vi "real time imaging v1.vi"() -> ()   [LabVIEW 2016]
uses:
  C:/Laser generated ultrasound/Labview/Kinesis Control/Thorlabs.MotionControl.Controls.dll
  Thorlabs.MotionControl.Controls.dll
  C:/Laser generated ultrasound/Labview/Kinesis Control/Thorlabs.MotionControl.KCube.BrushlessMotorCLI.dll
  Thorlabs.MotionControl.KCube.BrushlessMotorCLI.dll
  <vilib>/Analysis/3filter.llb/Filter Passband Type.ctl
  <vilib>/Analysis/baseanly.llb/Mean (DBL).vi
  <vilib>/Analysis/baseanly.llb/Real A x B.vi
  <vilib>/Utility/file.llb/Write To Spreadsheet File (DBL).vi
  <instrlib>/niScope/Acquire/Fetch/niScope Fetch.vi
  <vilib>/Analysis/Matrix/Numeric/Conversions/Array To Matrix - RA2.vi
  <vilib>/Analysis/Matrix/Numeric/Conversions/Matrix To Array - RM.vi
  <vilib>/Analysis/3filter.llb/Butterworth Filter (DBL).vi
  <instrlib>/niScope/Acquire/Fetch/niScope Multi Fetch.vi
  <vilib>/Analysis/NI_AALBase.lvlib
  <vilib>/Analysis/Matrix/NI_Matrix.lvlib
  <vilib>/Analysis/NI_AALPro.lvlib
panel:
  in  "stop":bool
  in  "Tab Control":T1(tab)
  in  "File Location":string="C:\\Laser generated ultrasound\\Labview\\Kinesis Control\\test data"
  in  "File name":string="scan_1"
  in  "SerialNumber":string="28251512"
  in  "Scan Length (mm)":dbl=20.0
  in  "Pullback speed (mm/s)":dbl=40.0
  in  "Repetition rate (Hz)":dbl=100.0
  in  "vertical range (V)":dbl=0.5 min=0.0 max=10.0 step=0.5
  in  "Depth (mm)":i32=15
  in  "Start acquisition":bool
  out "Number of samples":dbl
  out "number of a-lines":dbl
  in  "Apply frequency filter":bool
  in  "High Cutoff (MHz)":dbl=45.0
  in  "Low Cutoff (MHz)":dbl=1.0
  in  "Number of points":i32=150
  in  "Exponent":dbl=2.5
  out "?":cluster{dbl[], dbl[]}(graph)
  in  "Preview A-line?":bool
  in  "Start save":bool
  out "Intensity Graph":dbl[][](graph)
  in  "Stop save":bool
  out "Acquiring Data":bool
  in  "KCubeBrushlessControl":refnum<k24>(container)
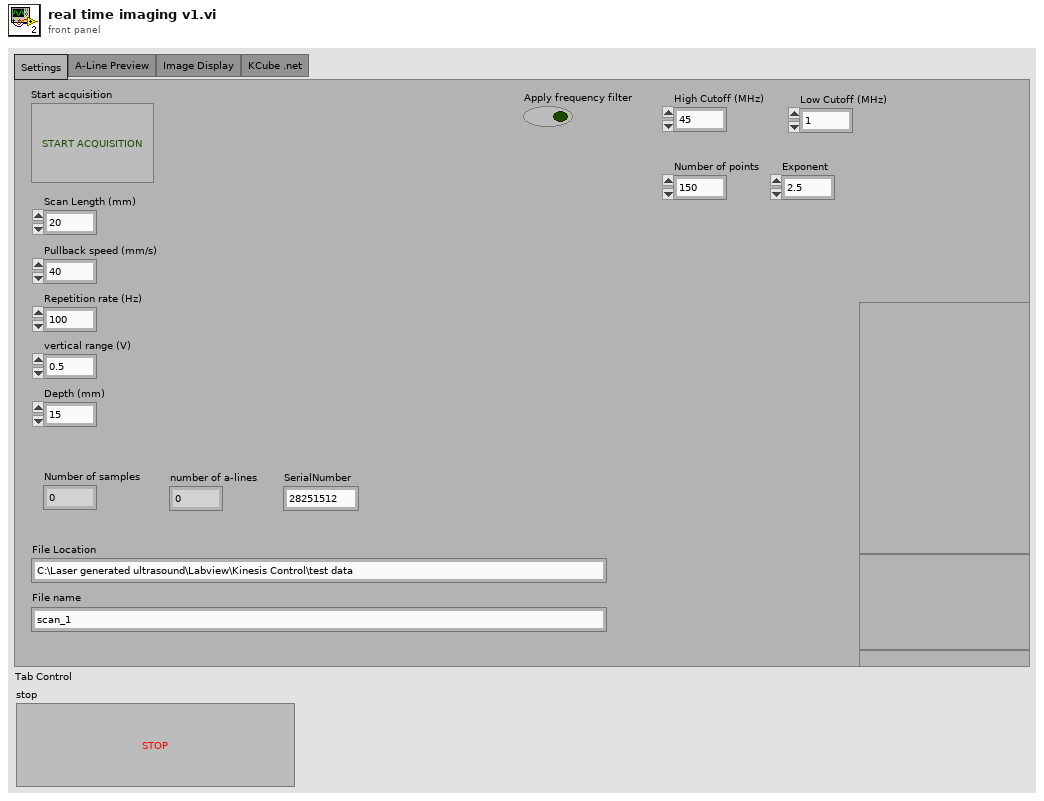
[diagram p1: front panel]
types:
  T1 = enum32{"Settings", "A-Line Preview", "Image Display", "KCube .net"}
  T2 = typedef "NI_AALBase.lvlib/Filter Passband Type.ctl" = enum32{"Lowpass", "Highpass", "Bandpass", "Bandstop"}
  T3 = typedef "NI_Matrix.lvlib/RealMatrix.ctl" = dbl[][]
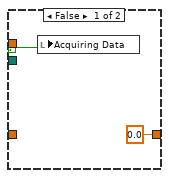
[diagram p8: hidden frame]
diagram:
  n1 = flat-sequence {
    tunnel: [w112] -> w71
    tunnel: [w111] -> w69
    tunnel: [w110] -> w67
    tunnel: [w108] -> w65
    tunnel: [w107] -> w63
    tunnel: [w95] -> w61
    tunnel: [w96] -> w59
    tunnel: ["Scan Length (mm)"] -> w57
    tunnel: ["Pullback speed (mm/s)"] -> w55
    tunnel: [w79] -> w53
    tunnel: ["File Location"] -> w52
    tunnel: ["File name"] -> w51
    tunnel: [w88] -> w43
    tunnel: [w88] -> w40
    tunnel: [w81] -> w10
    tunnel: ["Depth (mm)"] -> w5
    tunnel: [w79] -> w4
    tunnel: [w74] -> w3
    tunnel: [w73] -> w2
    tunnel: [w72] -> w1
    tunnel: w71 -> [w175]
    tunnel: [w175] -> w70
    tunnel: w69 -> [w174]
    tunnel: [w174] -> w68
    tunnel: w67 -> [w173]
    tunnel: [w173] -> w66
    tunnel: w65 -> [w172]
    tunnel: [w172] -> w64
    tunnel: w63 -> [w171]
    tunnel: [w171] -> w62
    tunnel: w61 -> [w170]
    tunnel: [w170] -> w60
    tunnel: w59 -> [w169]
    tunnel: [w169] -> w58
    tunnel: w57 -> [w168]
    tunnel: [w168] -> w56
    tunnel: w55 -> [w167]
    tunnel: [w167] -> w54
    tunnel: w53 -> [w165]
    tunnel: w52 -> [w135]
    tunnel: w51 -> [w134]
    tunnel: w43 -> [w142]
    tunnel: [w142] -> w42
    tunnel: w40 -> [w140]
    tunnel: w10 -> [_]
    tunnel: [w128] -> w9
    tunnel: w5 -> [w132]
    tunnel: w4 -> [w131]
    tunnel: w3 -> [w127]
    tunnel: w2 -> [w126]
    tunnel: w1 -> [w125]
    tunnel: w70 -> [w188]
    tunnel: w68 -> [w183]
    tunnel: w66 -> [w184]
    tunnel: [w188] -> w50
    tunnel: [w183] -> w49
    tunnel: [w184] -> w48
    tunnel: w64 -> [w182]
    tunnel: w62 -> [w181]
    tunnel: [w182] -> w47
    tunnel: [w181] -> w46
    tunnel: [w180] -> w45
    tunnel: w60 -> [w179]
    tunnel: [w179] -> w44
    tunnel: w58 -> [w180]
    tunnel: w56 -> [_]
    tunnel: w54 -> [w178]
    tunnel: w42 -> [w177]
    tunnel: [w177] -> w41
    tunnel: w9 -> [w176]
    tunnel: [w176] -> w8
    tunnel: w50 -> [w201]
    tunnel: [w201] -> w39
    tunnel: w49 -> [w200]
    tunnel: [w200] -> w37
    tunnel: w48 -> [w199]
    tunnel: [w199] -> w35
    tunnel: w47 -> [w198]
    tunnel: [w197] -> w33
    tunnel: w46 -> [w196]
    tunnel: [w195] -> w31
    tunnel: w45 -> [w194]
    tunnel: [w191] -> w29
    tunnel: w44 -> [w193]
    tunnel: [w190] -> w27
    tunnel: w41 -> [w192]
    tunnel: w8 -> [w189]
    tunnel: [w189] -> w7
    tunnel: w39 -> [w231]
    tunnel: [w231] -> w38
    tunnel: w37 -> [w230]
    tunnel: [w230] -> w36
    tunnel: w35 -> [w229]
    tunnel: [w229] -> w34
    tunnel: w33 -> [w228]
    tunnel: [w228] -> w32
    tunnel: w31 -> [w227]
    tunnel: [w227] -> w30
    tunnel: w29 -> [w226]
    tunnel: [w224] -> w28
    tunnel: w27 -> [w225]
    tunnel: [w223] -> w26
    tunnel: [w219] -> w25
    tunnel: w7 -> [w218]
    tunnel: [w218] -> w6
    tunnel: w38 -> [w243]
    tunnel: w36 -> [w241]
    tunnel: w34 -> [w242]
    tunnel: [w243] -> w24
    tunnel: [w241] -> w22
    tunnel: [w242] -> w20
    tunnel: w32 -> [w240]
    tunnel: w30 -> [w239]
    tunnel: [w240] -> w18
    tunnel: [w239] -> w16
    tunnel: [w235] -> w14
    tunnel: [w234] -> w12
    tunnel: w28 -> [w238]
    tunnel: w26 -> [w237]
    tunnel: w25 -> [w236]
    tunnel: w6 -> [w233]
    tunnel: w24 -> [w526]
    tunnel: [w526] -> w23
    tunnel: w22 -> [w525]
    tunnel: [w525] -> w21
    tunnel: w20 -> [w524]
    tunnel: [w524] -> w19
    tunnel: w18 -> [w523]
    tunnel: [w523] -> w17
    tunnel: w16 -> [w522]
    tunnel: [w522] -> w15
    tunnel: w14 -> [w521]
    tunnel: [w521] -> w13
    tunnel: w12 -> [w520]
    tunnel: [w520] -> w11
    tunnel: w23 -> [w528]
    tunnel: w21 -> [w527]
    tunnel: w19 -> [_]
    tunnel: w17 -> [w532]
    tunnel: w15 -> [w531]
    tunnel: w13 -> [w530]
    tunnel: w11 -> [w529]
    frame #0 {
      # "add extra a-lines as a buffer"
      # "calculate number of a-lines"
      # "Initiialise data array"
      # "round trip"
      # "speed of sound"
      # "convert depth to samples"
      # "convert to metre"
      # "Intialise all the equipment\n1. Motor\n2. Trigger\n3. Acquisition"
      n2 = Multiply(x=1500 ("y"), y=1e-08) -> (x*y=w100:dbl)
      n3 = local read "Pullback speed (mm/s)"() -> (w85:dbl)
      n4 = local read "Scan Length (mm)"() -> (w86:dbl)
      n5 = call "pulse_init.vi"("Repetition rate"="Repetition rate (Hz)") -> ("error out"=w107:errorcluster, "Refnum out"=w108:refnum<k21>)  [unwired: 9 in]
      n6 = local read "Repetition rate (Hz)"() -> (w84:dbl)
      n7 = Divide(x="Depth (mm)", y=1000) -> (x/y=w99:dbl)
      n8 = Multiply(x=w99, y=2.0) -> (x*y=w97:dbl)
      n9 = property class="KCubeBrushlessControl"(reference="KCubeBrushlessControl", "SerialNumber"="SerialNumber") -> (reference out=w116:refnum<k24>, error out=w115:errorcluster)  [unwired: 1 in]
      n10 = Divide(x=w97, y=w100) -> (x/y=w102:dbl)
      n11 = local read "Scan Length (mm)"() -> (w75:dbl)
      n12 = local read "Pullback speed (mm/s)"() -> (w73:dbl)
      n13 = Round Toward +Infinity(x=w102) -> (ceil(x): smallest int >= x=w79:dbl)
      "Number of samples" <- w79
      n14 = Initialize Array(0.0 ("element"), w79) -> (w89:dbl[])
      n15 = for {
        N: w79 -> [_]
        shift-right: [w124] -> w88
        shift-left: w89 -> [w123]
        i -> [w122]
        # "Create time axis"
        n16 = To Double Precision Float(number=w122) -> (double precision float=w121:dbl)
        n17 = Multiply(x=w121, y=1e-08) -> (x*y=w119:dbl)
        n18 = Replace Array Subset(array=w123, new element=w119, index=w122) -> (w124:dbl[])
      }
      n19 = Divide(x=w86, y=w85) -> (x/y=w83:dbl)
      n20 = local read "Repetition rate (Hz)"() -> (w72:dbl)
      n21 = Multiply(x=w83, y=w84) -> (x*y=w82:dbl)
      n22 = call "scope_init.vi"("Num Samples"=w79, "vertical range"="vertical range (V)", "Averages"=1) -> ("error out"=w95:errorcluster, "IVI Refnum out"=w96:refnum<k15>)  [unwired: 7 in]
      n23 = Initialize Array(0.0 ("element"), w79, w82) -> (w81:dbl[][])
      n24 = invoke class="KCubeBrushlessControl" method="CreateDevice"(reference=w116, error in=w115) -> (reference out=w114:refnum<k24>, error out=w113:errorcluster)  [unwired: 1 in, 1 out]
      n25 = Divide(x=w73, y=w72) -> (x/y=w76:dbl)
      n26 = Divide(x=w75, y=w76) -> (x/y=w77:dbl)
      n27 = Add(x=w77, y=0.0) -> (x+y=w74:dbl)
      "number of a-lines" <- w74
      n28 = property class="KCubeBrushlessControl"(reference=w114, error in=w113) -> (reference out=w112:refnum<k24>, error out=w111:errorcluster, "Device"=w110:refnum<k24>)
    }
    frame #1 {
      w143 = "\r"
      w146 = "\t"
      # "Save the header file"
      # "Initialise the data matrix"
      # "Initialise the data matrix\nSave the Header file"
      n29 = local read "Repetition rate (Hz)"() -> (w152:dbl)
      n30 = local read "Number of samples"() -> (w158:dbl)
      n31 = local read "number of a-lines"() -> (w155:dbl)
      n32 = local read "Scan Length (mm)"() -> (w149:dbl)
      n33 = local read "Pullback speed (mm/s)"() -> (w145:dbl)
      n34 = Number To Decimal String(number=w158) -> (decimal integer string=w157:string)  [unwired: 1 in]
      n35 = Number To Decimal String(number=w152) -> (decimal integer string=w151:string)  [unwired: 1 in]
      n36 = Number To Decimal String(number=w155) -> (decimal integer string=w154:string)  [unwired: 1 in]
      n37 = Number To Decimal String(number=w149) -> (decimal integer string=w148:string)  [unwired: 1 in]
      n38 = Concatenate Strings(w135, "\\" ("string"), w134, "_hdr.txt" ("string")) -> (w163:string)
      n39 = Divide(x=w132, y=w131) -> (x/y=w130:dbl)
      n40 = Number To Decimal String(number=w145) -> (decimal integer string=w144:string)  [unwired: 1 in]
      n41 = Concatenate Strings(w135, "\\" ("string"), w134, "_taxis.txt" ("string")) -> (w139:string)
      n42 = Divide(x=w126, y=w125) -> (x/y=w133:dbl)
      n43 = String To Path(string=w139) -> (path=w136:path)
      n44 = property on="Intensity Graph" class="IntGraph (strict)"("XScale.Multiplier"=w133, "YScale.Multiplier"=w130) -> ()  [unwired: 2 in, 2 out]
      n45 = property on="Intensity Graph" class="IntGraph (strict)"("ZScale.MarkerVals[]"=cluster{dbl, u32}[] [{0.0, 0}, {25.0, 16711680}, {50.0, 16744192}, {75.0, 16777087}, {100.0, 16777215}] ("Z Scale.Marker Values[]")) -> ()  [unwired: 2 in, 2 out]
      n46 = Initialize Array(0.0 ("element"), w165, w127) -> (w128:dbl[][])
      n47 = call-poly <vilib>:"Write To Spreadsheet File.vi"("format (%.3f)"="%#g", "1D data"=w140, "file path (dialog if empty)"=w136) -> ()  [unwired: 5 in, 1 out]
      n48 = Concatenate Strings("Samples per A-line" ("string"), w146, w157, w143, "Number of A-lines" ("string"), w146, w154, w143, "Repetition rate (Hz)" ("string"), w146, w151, w143, "Scan length (mm)" ("string"), w146, w148, w143, "Pullback speed (mm/s)" ("string"), w146, w144, w143) -> (w160:string)
      n49 = String To Path(string=w163) -> (path=w164:path)
      n50 = Write to Text File(file (use dialog)=w164, text=w160) -> ()  [unwired: 2 in, 3 out]
    }
    frame #2 {
      # "Initial data array"
      # "Home the motor"
      n51 = invoke class="KCubeBrushlessMotor" method="Home"(reference=w184, error in=w183, "waitTimeout"=50000) -> ()  [unwired: 1 in, 4 out]
      n52 = invoke class="KCubeBrushlessMotor" method="SetVelocityParams"(reference=w184, error in=w183, "maxVelocity"=w178, "acceleration"=999.7) -> ()  [unwired: 1 in, 5 out]
      n53 = Wait (ms)(milliseconds to wait=u32 1000) -> ()  [unwired: 1 out]
    }
    frame #3 {
      # "A-line display for positioning"
      n54 = while {
        tunnel: w198 -> [w216]
        tunnel: w196 -> [w215]
        tunnel: [w216] -> w197
        tunnel: [w215] -> w195
        tunnel: w194 -> [w212]
        tunnel: w193 -> [w211]
        tunnel: w192 -> [w206]
        tunnel: [w203] -> w191
        tunnel: [w202] -> w190
        stop <- "Start acquisition" stop-if-true
        n55 = local read "Number of samples"() -> (w214:dbl)
        n56 = call <instrlib>:"niScope Initiate Acquisition.vi"("instrument handle"=w212, "error in"=w211) -> ("instrument handle out"=w210:refnum<k15>, "error out"=w209:errorcluster)  [unwired: 12 in]
        n57 = call-poly <instrlib>:"niScope Fetch (poly).vi"("error in"=w209, "numSamples"=w214, "channels"="0", "instrument handle"=w210) -> ("error out"=w202:errorcluster, "wfm"=w208:dbl[], "instrument handle out"=w203:refnum<k15>)  [unwired: 4 in, 1 out]
        n58 = Bundle(w206, "wfm"=w208) -> (w207:cluster{dbl[], "wfm":dbl[]})  [unwired: 1 in]
        n59 = case shown="True" "Preview A-line?" {
          tunnel: w207 -> [_ w217]
          frame False {
          }
          frame True {
            "?" <- w217
          }
        }
      }
    }
    frame #4 {
      # "Setup acquisition cards to record all a-lines"
      n60 = local read "Number of samples"() -> (w219:dbl)
      n61 = local read "number of a-lines"() -> (w220:dbl)
      n62 = call <instrlib>:"niScope Configure Horizontal Timing.vi"("instrument handle"=w226, "number of records"=w220, "min sample rate"=100000000.0, "reference position"=0.0, "error in"=w225, "min record length"=w219) -> ("instrument handle out"=w224:refnum<k15>, "error out"=w223:errorcluster)  [unwired: 8 in]
    }
    frame #5 {
      w232 = 0.0 ("y")
      # "move to end and acquire data\n1. move motor\n2. acquire data"
      n63 = while {
        tunnel: w242 -> [w285]
        tunnel: w241 -> [w284]
        tunnel: w236 -> [w281]
        shift-right: [w277] -> w235
        shift-left: w238 -> [w283]
        shift-right: [w276] -> w234
        shift-left: w237 -> [w282]
        shift-right: [w275] -> _
        shift-left: w233 -> [w274]
        shift-right: [w273] -> _
        shift-left: w232 -> [w272]
        shift-right: [w271] -> _
        shift-left: w232 -> [w270]
        shift-right: [w269] -> _
        shift-left: w232 -> [w268]
        stop <- "stop" stop-if-true
        # "Image number increment"
        # "Numeric to act as boolean to keep save going"
        n64 = call <instrlib>:"niScope Initiate Acquisition.vi"("instrument handle"=w283, "error in"=w282) -> ("instrument handle out"=w280:refnum<k15>, "error out"=w279:errorcluster)  [unwired: 12 in]
        n65 = flat-sequence {
          tunnel: w285 -> [w339]
          tunnel: w284 -> [w338]
          tunnel: w281 -> [w289]
          tunnel: w280 -> [w334]
          tunnel: w279 -> [w333]
          tunnel: [w337] -> w267
          tunnel: [w336] -> w265
          tunnel: [w286] -> w263
          tunnel: [w286] -> w261
          tunnel: [w329] -> w259
          tunnel: [w328] -> w257
          tunnel: w274 -> [w294]
          tunnel: [w286] -> w255
          tunnel: [w320] -> w253
          tunnel: w272 -> [w318]
          tunnel: w270 -> [w313]
          tunnel: [w312] -> w251
          tunnel: w268 -> [w311]
          tunnel: [w311] -> w249
          tunnel: ["Apply frequency filter"] -> w247
          tunnel: [w289] -> w245
          tunnel: w267 -> [w396]
          tunnel: [w394] -> w266
          tunnel: w265 -> [w395]
          tunnel: [w393] -> w264
          tunnel: w263 -> [w406]
          tunnel: [w406] -> w262
          tunnel: w261 -> [w405]
          tunnel: [w405] -> w260
          tunnel: w259 -> [w404]
          tunnel: [w404] -> w258
          tunnel: w257 -> [w403]
          tunnel: [w403] -> w256
          tunnel: w255 -> [w402]
          tunnel: [w402] -> w254
          tunnel: w253 -> [w401]
          tunnel: [w401] -> w252
          tunnel: w251 -> [w400]
          tunnel: [w400] -> w250
          tunnel: w249 -> [w399]
          tunnel: [w399] -> w248
          tunnel: w247 -> [w398]
          tunnel: [w398] -> w246
          tunnel: w245 -> [w397]
          tunnel: [w397] -> w244
          tunnel: [w449] -> w276
          tunnel: [w450] -> w277
          tunnel: w266 -> [w452]
          tunnel: w264 -> [w451]
          tunnel: w262 -> [w455]
          tunnel: w260 -> [w416]
          tunnel: w258 -> [w448]
          tunnel: w256 -> [w447]
          tunnel: w254 -> [w442]
          tunnel: [w407] -> w275
          tunnel: [w441] -> w273
          tunnel: w252 -> [w435]
          tunnel: w250 -> [w426]
          tunnel: [w439] -> w271
          tunnel: w248 -> [w434]
          tunnel: [w436] -> w269
          tunnel: w246 -> [w413]
          tunnel: w244 -> [w410]
          frame #0 {
            w297 = 20 ("length")
            # "Frequency filter"
            # "cross-talk removal"
            # "Calculate the running average"
            # "take first few A-lines to repeat and use for running average"
            # "0 - 2000 - time\n1 - 50 - a-lines"
            # "NEXT STEPS:\n\nWork on the timing for motor movements"
            n66 = local read "Scan Length (mm)"() -> (w330:dbl)
            n67 = local read "Number of samples"() -> (w298:dbl)
            n68 = Number To Decimal String(number=w311) -> (decimal integer string=w310:string)  [unwired: 1 in]
            n69 = Number To Decimal String(number=w318) -> (decimal integer string=w308:string)  [unwired: 1 in]
            n70 = local read "File Location"() -> (w323:string)
            n71 = local read "File name"() -> (w321:string)
            n72 = invoke class="KCubeBrushlessMotor" method="MoveTo"(reference=w339, error in=w338, "position"=w330, "waitTimeout"=2000) -> (reference out=w329:refnum<k24>, error out=w328:errorcluster)  [unwired: 1 in, 3 out]
            n73 = Array Subset(array=w294, index (row)=0 ("index"), length (row)=w298, index (col)=0 ("index"), length (col)=w297) -> (w301:dbl[][])
            n74 = Concatenate Strings(w323, "\\" ("string"), w321, "_image_" ("string"), w310, "_f_" ("string"), w308, ".txt" ("string")) -> (w325:string)
            n75 = for {
              tunnel: w301 -> [w385] mode=indexing
              tunnel: [w384] -> w300 mode=indexing
              n76 = Reverse 1D Array(array=w385) -> (reversed array=w384:dbl[])
            }
            n77 = call-poly <instrlib>:"niScope Fetch (poly).vi"("timeout"=-1.0, "error in"=w333, "numSamples"=w289, "channels"="0", "instrument handle"=w334) -> ("error out"=w336:errorcluster, "wfm"=w305:dbl[][], "instrument handle out"=w337:refnum<k15>)  [unwired: 3 in, 1 out]
            n78 = String To Path(string=w325) -> (path=w324:path)
            n79 = Equal?(x=w313, y=1.0) -> (x = y?=w315:bool)
            n80 = Or(x="Start save", y=w315) -> (x .or. y?=w317:bool)
            n81 = local read "number of a-lines"() -> (w296:dbl)
            n82 = Insert Into Array(array=w294, index (col)=0 ("disabled index (col)"), new element=w300) -> (w299:dbl[][])  [unwired: 1 in]
            n83 = case shown="True" w317 {
              tunnel: w294 -> [_ w391]
              tunnel: w324 -> [_ w390]
              tunnel: [w388 w389] -> w320
              tunnel: w318 -> [w388 w389]
              frame False {
              }
              frame True {
                n84 = call-poly <vilib>:"Write To Spreadsheet File.vi"("format (%.3f)"="%#g", "2D data"=w391, "file path (dialog if empty)"=w390) -> ()  [unwired: 5 in, 1 out]
              }
            }
            n85 = for {
              N: w296 -> [_]
              tunnel: w299 -> [w381]
              tunnel: w298 -> [w379]
              tunnel: w297 -> [w377]
              tunnel: [w375] -> w295 mode=indexing
              i -> [w378]
              n86 = Array Subset(array=w381, index (row)=0 ("index"), length (row)=w379, index (col)=w378, length (col)=w377) -> (w376:dbl[][])
              n87 = for {
                tunnel: w376 -> [w383] mode=indexing
                tunnel: [w382] -> w375 mode=indexing
                n88 = call-poly <vilib>:"Mean.vi"("X"=w383) -> ("mean"=w382:dbl)  [unwired: 1 out]
              }
            }
            n89 = Transpose 2D Array(2D array=w305) -> (transposed array=w287:dbl[][])
            n90 = case shown="True" "Start save" {
              tunnel: w313 -> [w386 _]
              tunnel: [w386 1.0 ("y")] -> w312
              frame False {
              }
              frame True {
              }
            }
            n91 = Transpose 2D Array(2D array=w294) -> (transposed array=w293:dbl[][])
            n92 = Replace Array Subset(array=w294, new element=w287, index (row)=0, index (col)=0 ("disabled index (col)")) -> (w286:dbl[][])
            n93 = for {
              N: w296 -> [_]
              tunnel: w295 -> [w368] mode=indexing
              tunnel: w293 -> [w367] mode=indexing
              tunnel: [w365] -> w292 mode=indexing
              n94 = call "create_design_matrix.vi"("input vector"=w368) -> ("design matrix"=w374:dbl[][])
              n95 = Array Size(array=w367) -> (size(s)=w369:i32)
              n96 = call "linear_fit.vi"("Real 1D Array"=w367, "X"=w374) -> ("A x B"=w373:T3)
              n97 = call-poly <vilib>:"Array To Matrix.vi"("Real 2D Array"=w374) -> ("Real Matrix"=w372:T3)
              n98 = call-poly <vilib>:"A x B.vi"("B"=w372, "A"=w373) -> ("A x B"=w371:T3)  [unwired: 1 out]
              n99 = call-poly <vilib>:"Matrix To Array.vi"("Real Matrix"=w371) -> ("Real 2D Array"=w370:dbl[][])
              n100 = Reshape Array(w370, w369) -> (w366:dbl[])
              n101 = Subtract(x=w367, y=w366) -> (x-y=w365:dbl[])
            }
            n102 = Wait (ms)(milliseconds to wait=u32 5) -> ()  [unwired: 1 out]
            n103 = case shown="True" "Apply frequency filter" {
              tunnel: w292 -> [w347 w349]
              tunnel: [w347 w348] -> w291
              frame False {
              }
              frame True {
                n104 = Multiply(x="High Cutoff (MHz)", y=1000000.0) -> (x*y=w355:dbl)
                n105 = Multiply(x="Low Cutoff (MHz)", y=1000000.0) -> (x*y=w354:dbl)
                n106 = for {
                  tunnel: 100000000.0 ("y") -> [w361]
                  tunnel: w355 -> [w360]
                  tunnel: w354 -> [w359]
                  tunnel: w349 -> [w358] mode=indexing
                  tunnel: [w357] -> w348 mode=indexing
                  n107 = call-poly <vilib>:"Butterworth Filter.vi"("init/cont (init:F)"=FALSE, "order"=8, "filter type"=Filter_Passband_Type."Bandpass", "low cutoff freq: fl"=w359, "high cutoff freq: fh"=w360, "sampling freq: fs"=w361, "X"=w358) -> ("Filtered X"=w357:dbl[])  [unwired: 1 in, 1 out]
                }
              }
            }
            n108 = for {
              tunnel: w291 -> [w346] mode=indexing
              tunnel: [w340] -> w288 mode=indexing
              n109 = call <vilib>:"Fast Hilbert Transform.vi"("X"=w346) -> ("Hilbert{X}"=w345:dbl[])  [unwired: 1 out]
              n110 = Absolute Value(x=w345) -> (abs(x)=w344:dbl[])
              n111 = call "TGC_exponential.vi"("Exponent"="Exponent", "Number of points"="Number of points", "Input vector"=w344) -> ("Output vector"=w341:dbl[])
              n112 = Logarithm Base 10(1:w341) -> (0:w340:dbl[])
            }
            n113 = local write "Intensity Graph"(w288) -> ()
          }
          frame #1 {
            n114 = call <instrlib>:"niScope Initiate Acquisition.vi"("instrument handle"=w396, "error in"=w395) -> ("instrument handle out"=w394:refnum<k15>, "error out"=w393:errorcluster)  [unwired: 12 in]
          }
          frame #2 {
            w421 = 20 ("length")
            # "Frequency filter"
            # "cross-talk removal"
            # "Calculate the running average"
            n115 = local read "File name"() -> (w456:string)
            n116 = local read "File Location"() -> (w457:string)
            n117 = Number To Decimal String(number=w434) -> (decimal integer string=w432:string)  [unwired: 1 in]
            n118 = Number To Decimal String(number=w435) -> (decimal integer string=w430:string)  [unwired: 1 in]
            n119 = invoke class="KCubeBrushlessMotor" method="MoveTo"(reference=w448, error in=w447, "position"=0.0, "waitTimeout"=2000) -> ()  [unwired: 1 in, 5 out]
            n120 = Concatenate Strings(w457, "\\" ("string"), w456, "_image_" ("string"), w432, "_b_" ("string"), w430, ".txt" ("string")) -> (w460:string)
            n121 = local read "Number of samples"() -> (w420:dbl)
            n122 = String To Path(string=w460) -> (path=w458:path)
            n123 = call-poly <instrlib>:"niScope Fetch (poly).vi"("timeout"=-1.0, "error in"=w451, "numSamples"=w410, "channels"="0", "instrument handle"=w452) -> ("error out"=w449:errorcluster, "wfm"=w427:dbl[][], "instrument handle out"=w450:refnum<k15>)  [unwired: 3 in, 1 out]
            n124 = Equal?(x=1.0, y=w426) -> (x = y?=w438:bool)
            n125 = case shown="True" w438 {
              selector: w438 -> [w512 w514]
              tunnel: w455 -> [_ w518]
              tunnel: w458 -> [_ w517]
              tunnel: w435 -> [_ w516]
              tunnel: [0.0 w515] -> w441
              frame False {
                n126 = local write "Acquiring Data"(w512) -> ()
              }
              frame True {
                n127 = call-poly <vilib>:"Write To Spreadsheet File.vi"("format (%.3f)"="%#g", "2D data"=w518, "file path (dialog if empty)"=w517) -> ()  [unwired: 5 in, 1 out]
                n128 = Increment(x=w516) -> (x+1=w515:dbl)
                "Acquiring Data" <- w514
              }
            }
            n129 = Array Subset(array=w416, index (row)=0 ("index"), length (row)=w420, index (col)=0 ("index"), length (col)=w421) -> (w419:dbl[][])
            n130 = Transpose 2D Array(2D array=w427) -> (transposed array=w408:dbl[][])
            n131 = for {
              tunnel: w419 -> [w497] mode=indexing
              tunnel: [w496] -> w418 mode=indexing
              n132 = Reverse 1D Array(array=w497) -> (reversed array=w496:dbl[])
            }
            n133 = local read "number of a-lines"() -> (w411:dbl)
            n134 = Wait (ms)(milliseconds to wait=u32 5) -> ()  [unwired: 1 out]
            n135 = Insert Into Array(array=w416, index (col)=0 ("disabled index (col)"), new element=w418) -> (w422:dbl[][])  [unwired: 1 in]
            n136 = for {
              N: w411 -> [_]
              tunnel: w422 -> [w504]
              tunnel: w420 -> [w502]
              tunnel: w421 -> [w500]
              tunnel: [w498] -> w417 mode=indexing
              i -> [w501]
              n137 = Array Subset(array=w504, index (row)=0 ("index"), length (row)=w502, index (col)=w501, length (col)=w500) -> (w499:dbl[][])
              n138 = for {
                tunnel: w499 -> [w506] mode=indexing
                tunnel: [w505] -> w498 mode=indexing
                n139 = call-poly <vilib>:"Mean.vi"("X"=w506) -> ("mean"=w505:dbl)  [unwired: 1 out]
              }
            }
            n140 = case shown="True" "Stop save" {
              tunnel: w426 -> [w508 _]
              tunnel: [w508 0.0 ("y")] -> w439
              tunnel: w434 -> [w507 w510]
              tunnel: [w507 w509] -> w436
              frame False {
              }
              frame True {
                n141 = Increment(x=w510) -> (x+1=w509:dbl)
              }
            }
            n142 = Transpose 2D Array(2D array=w416) -> (transposed array=w415:dbl[][])
            n143 = Replace Array Subset(array=w442, new element=w408, index (row)=0, index (col)=0 ("disabled index (col)")) -> (w407:dbl[][])
            n144 = for {
              N: w411 -> [_]
              tunnel: w417 -> [w489] mode=indexing
              tunnel: w415 -> [w488] mode=indexing
              tunnel: [w486] -> w414 mode=indexing
              n145 = call "create_design_matrix.vi"("input vector"=w489) -> ("design matrix"=w495:dbl[][])
              n146 = Array Size(array=w488) -> (size(s)=w490:i32)
              n147 = call "linear_fit.vi"("Real 1D Array"=w488, "X"=w495) -> ("A x B"=w494:T3)
              n148 = call-poly <vilib>:"Array To Matrix.vi"("Real 2D Array"=w495) -> ("Real Matrix"=w493:T3)
              n149 = call-poly <vilib>:"A x B.vi"("B"=w493, "A"=w494) -> ("A x B"=w492:T3)  [unwired: 1 out]
              n150 = call-poly <vilib>:"Matrix To Array.vi"("Real Matrix"=w492) -> ("Real 2D Array"=w491:dbl[][])
              n151 = Reshape Array(w491, w490) -> (w487:dbl[])
              n152 = Subtract(x=w488, y=w487) -> (x-y=w486:dbl[])
            }
            n153 = case shown="True" w413 {
              tunnel: w414 -> [w468 w472]
              tunnel: [w468 w471] -> w412
              frame False {
              }
              frame True {
                n154 = local read "High Cutoff (MHz)"() -> (w470:dbl)
                n155 = local read "Low Cutoff (MHz)"() -> (w469:dbl)
                n156 = Multiply(x=w470, y=1000000.0) -> (x*y=w476:dbl)
                n157 = Multiply(x=w469, y=1000000.0) -> (x*y=w475:dbl)
                n158 = for {
                  tunnel: 100000000.0 ("y") -> [w482]
                  tunnel: w476 -> [w481]
                  tunnel: w475 -> [w480]
                  tunnel: w472 -> [w479] mode=indexing
                  tunnel: [w478] -> w471 mode=indexing
                  n159 = call-poly <vilib>:"Butterworth Filter.vi"("init/cont (init:F)"=FALSE, "order"=8, "filter type"=Filter_Passband_Type."Bandpass", "low cutoff freq: fl"=w480, "high cutoff freq: fh"=w481, "sampling freq: fs"=w482, "X"=w479) -> ("Filtered X"=w478:dbl[])  [unwired: 1 in, 1 out]
                }
              }
            }
            n160 = for {
              tunnel: w412 -> [w467] mode=indexing
              tunnel: [w463] -> w409 mode=indexing
              n161 = local read "Number of points"() -> (w462:i32)
              n162 = call <vilib>:"Fast Hilbert Transform.vi"("X"=w467) -> ("Hilbert{X}"=w466:dbl[])  [unwired: 1 out]
              n163 = local read "Exponent"() -> (w461:dbl)
              n164 = Absolute Value(x=w466) -> (abs(x)=w465:dbl[])
              n165 = call "TGC_exponential.vi"("Exponent"=w461, "Number of points"=w462, "Input vector"=w465) -> ("Output vector"=w464:dbl[])
              n166 = Logarithm Base 10(1:w464) -> (0:w463:dbl[])
            }
            n167 = local write "Intensity Graph"(w409) -> ()
          }
        }
      }
    }
    frame #6 {
      # "Save data"
    }
    frame #7 {
      # "Close everything"
      n168 = call <vilib>:"DAQmx Stop Task.vi"("task/channels in"=w532, "error in"=w531) -> ("task out"=w534:refnum<k21>, "error out"=w533:errorcluster)  [unwired: 12 in]
      n169 = call <instrlib>:"niScope Close.vi"("instrument handle"=w530, "error in"=w529) -> ()  [unwired: 13 in, 1 out]
      n170 = call <vilib>:"DAQmx Clear Task.vi"("task in"=w534, "error in"=w533) -> ()  [unwired: 13 in, 1 out]
      n171 = invoke class="KCubeBrushlessControl" method="CloseDevice"(reference=w528, error in=w527) -> ()  [unwired: 1 in, 3 out]
    }
  }
